vi "Event Messenger Channel Lesson 6.vi"() -> ()   [LabVIEW 2019]
doc: "Lesson 6 is the same messaging system as Lesson 5 but uses a LabVIEW class message hierarchy. This lesson shows the event channels in a form that is highly flexible for a multiple-module system. Its architecture is very similar to the Actor Framework. Channel wires express static connections between parallel systems; AF expresses dynamic connections."
uses:
  <extravilib>/ChannelInstances/Event Messenger-class'Draw Messages.lvlib-Draw Message'/Event Data.ctl
  SubVIs/Draw Messages/Draw Message/Draw Message.lvclass
  <extravilib>/ChannelInstances/Event Messenger-u32/Event Data.ctl
  SubVIs/Draw Messages/Reset Message/Reset Message.lvclass
  e:/builds/penguin/labview/branches/2019/dev/dist/examples/Channels/Event Messenger/SubVIs/Draw Messages/Draw Message/Draw Message.lvclass
  SubVIs/Draw Messages/Square Message/Square Message.lvclass
  SubVIs/Draw Messages/Circle Message/Circle Message.lvclass
  <extravilib>/ChannelInstances/Event Messenger-class'Draw Messages.lvlib-Draw Message'/Instantiate.vi
  <extravilib>/ChannelInstances/Event Messenger-class'Draw Messages.lvlib-Draw Message'/))Channel.vi
  <extravilib>/ChannelInstances/Event Messenger-u32/Instantiate.vi
  <extravilib>/ChannelInstances/Event Messenger-u32/))Channel.vi
  <extravilib>/ChannelInstances/Event Messenger-u32.lvlib
  <extravilib>/ChannelInstances/Event Messenger-class'Draw Messages.lvlib-Draw Message'.lvlib
panel:
  out "Picture":picture
  out "current color":u32(colorbox)
  out "command log":string
  in  "Stop Gamma":bool
  in  "Stop Epsilon":bool
  in  "Stop Beta":bool
  in  "Stop Alpha":bool
  # "Overview: This VI demonstrates how to use the Event Messenger channel wire.\n\nLesson 6 is the same messaging system as Lesson 5 but uses a LabVIEW class message hierarchy. This lesson uses the channels to form a flexible, multiple-module system. Its architecture is very similar to the Actor Framework. Channel wires express static connections between parallel systems; AF expresses dynamic connections.\n\nInstructions:\n1. Run the VI. There are three producers and two consumers, all running at various speeds. Alpha and beta loops produce object commands. Gamma loop produces a color. Delta loop has the job to log all the commands. Epsilon loop actually does the work of the commands and handles color changes. Epsilon also sends commands to itself, which are properly logged by Delta.\n\n2. Stop the VI by pressing any of the STOP buttons. There will be a slight delay until loop Gamma stops because of its 2 second Wait. \n\n3. Open the block diagram. Review the comments there to see how this VI works."
  # "Producers"
  # "Consumers"
  # "Consumer Delta"
  # "Consumer Epsilon"
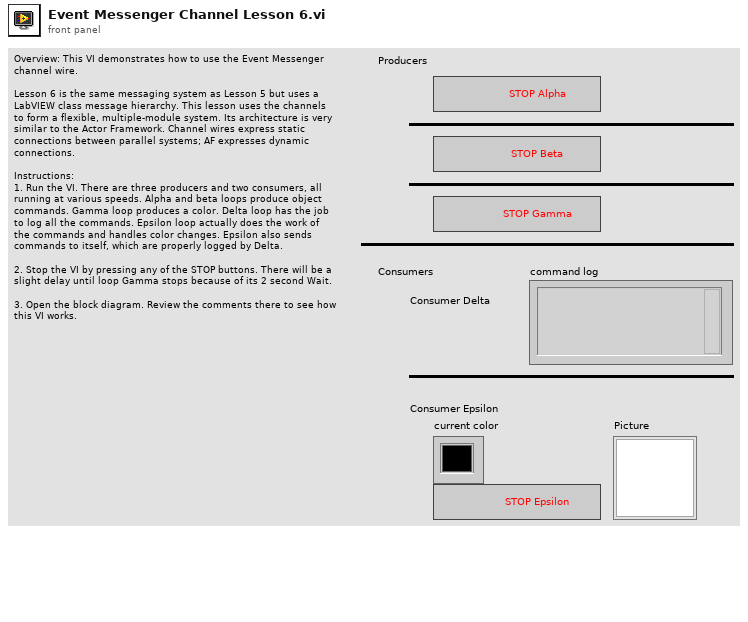
[diagram p1: front panel]
types:
  T1 = cluster{"command":refnum<event-registration>, "new color":refnum<event-registration>}
  T2 = typedef "Event Messenger-class'Draw Messages.lvlib-Draw Message'.lvlib/))Channel.ctl" = refnum<queue>
  T3 = typedef "Event Messenger-u32.lvlib/))Channel.ctl" = refnum<queue>
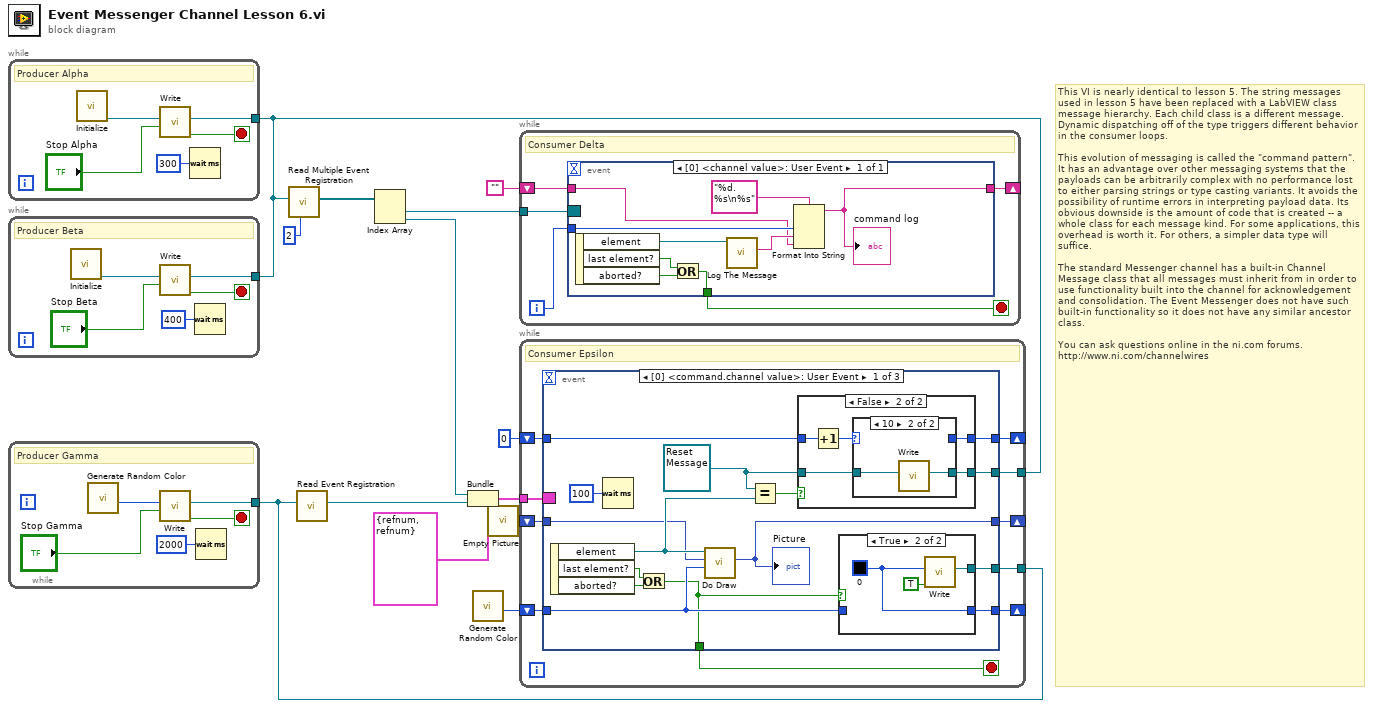
[diagram p0: block diagram]
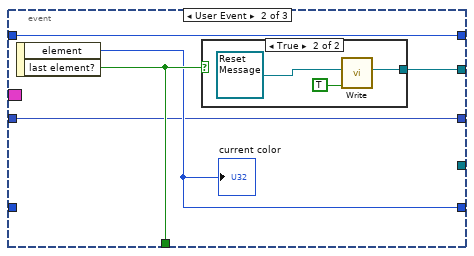
[diagram p5: hidden frame]
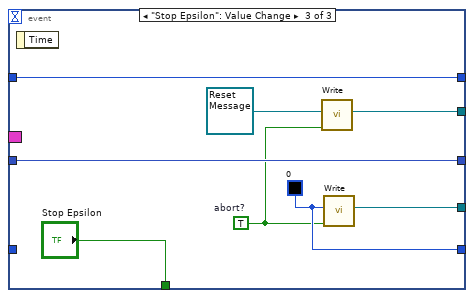
[diagram p7: hidden frame]
diagram:
  # "This VI is nearly identical to lesson 5. The string messages used in lesson 5 have been replaced with a LabVIEW class message hierarchy. Each child class is a different message. Dynamic dispatching off of the type triggers different behavior in the consumer loops.\n\nThis evolution of messaging is called the \"command pattern\". It has an advantage over other messaging systems that the payloads can be arbitrarily complex with no performance lost to either parsing strings or type casting variants. It avoids the possibility of runtime errors in interpreting payload data. Its obvious downside is the amount of code that is created -- a whole class for each message kind. For some applications, this overhead is worth it. For others, a simpler data type will suffice.\n\nThe standard Messenger channel has a built-in Channel Message class that all messages must inherit from in order to use functionality built into the channel for acknowledgement and consolidation. The Event Messenger does not have such built-in functionality so it does not have any similar ancestor class.\n\nYou can ask questions online in the ni.com forums. \nhttp://www.ni.com/channelwires"
  n1 = while {
    tunnel: [w18] -> w2
    stop <- w16 stop-if-true
    # "Producer Alpha"
    n2 = call "Initialize.vi"() -> ("Draw Message"=w14:refnum<class "Draw Message.lvclass">)  [unwired: 11 in]
    n3 = call <extravilib>:"Write.vi"("last element? (F)"="Stop Alpha", "element"=w14) -> ("done?"=w16:bool, "channel"=w18:T2)  [unwired: 8 in]
    n4 = Wait (ms)(milliseconds to wait=u32 300) -> ()  [unwired: 1 out]
  }
  n5 = while {
    tunnel: w2 -> [w21]
    stop <- w22 stop-if-true
    # "Producer Beta"
    n6 = call "Initialize.vi"() -> ("Draw Message"=w19:refnum<class "Draw Message.lvclass">)  [unwired: 7 in]
    n7 = call <extravilib>:"Write.vi"("last element? (F)"="Stop Beta", "element"=w19) -> ("done?"=w22:bool, "channel"=w21:T2)  [unwired: 8 in]
    n8 = Wait (ms)(milliseconds to wait=u32 400) -> ()  [unwired: 1 out]
  }
  n9 = while {
    tunnel: [w26] -> w7
    stop <- w27 stop-if-true
    # "Producer Gamma"
    n10 = call "Generate Random Color.vi"() -> ("Color"=w24:u32)  [unwired: 11 in]
    n11 = call <extravilib>:"Write.vi"("last element? (F)"="Stop Gamma", "element"=w24) -> ("done?"=w27:bool, "channel"=w26:T3)  [unwired: 8 in]
    n12 = Wait (ms)(milliseconds to wait=u32 2000) -> ()  [unwired: 1 out]
  }
  n13 = call <extravilib>:"Read Multiple Event Registration.vi"("number of event structures"=u16 2 ("# Event structures"), "channel"=w2) -> ("event registration refnums"=w10:refnum<event-registration>[])  [unwired: 9 in]
  n14 = call <extravilib>:"Read Event Registration.vi"("channel"=w7) -> ("event registration refnum"=w8:refnum<event-registration>)  [unwired: 10 in]
  n15 = Index Array(array=w10) -> (element #1=w12:refnum<event-registration>, element #2=w11:refnum<event-registration>)  [unwired: 2 in]
  n16 = Bundle(cluster=T1 {"command"=refnum, "new color"=refnum}, "command"=w11, "new color"=w8) -> (w13:T1)
  n17 = call "Generate Random Color.vi"() -> ("Color"=w6:u32)  [unwired: 11 in]
  n18 = call "Empty Picture"() -> ("empty picture"=w3:picture)
  n19 = while {
    tunnel: w12 -> [w33]
    shift-right: [w29] -> _
    shift-left: "" -> [w31]
    i -> [w30]
    stop <- w32 stop-if-true
    # "Consumer Delta"
    n20 = event shown="[0] <channel value>: User Event" {
      selector: w33 -> [_]
      dyn-events: _ -> [_]
      timeout: _ -> [_]
      tunnel: [w34] -> w32
      tunnel: w31 -> [w38]
      tunnel: w30 -> [w40]
      tunnel: [w37] -> w29
      event User Event {
        n21 = event-data() -> ("element"=w42:refnum<class "Draw Message.lvclass">, "last element?"=w35:bool, "aborted?"=w36:bool)  [unwired: 1 in]
        n22 = Or(x=w35, y=w36) -> (x .or. y?=w34:bool)
        n23 = call-dynamic "Log The Message.vi"("Draw Message"=w42) -> ("log text"=w39:string)  [unwired: 10 in]
        n24 = Format Into String(format string="%d. %s\n%s", w40, w39, w38) -> (resulting string=w37:string)  [unwired: 2 in, 1 out]
        "command log" <- w37
      }
    }
  }
  n25 = while {
    tunnel: w13 -> [w51]
    tunnel: w2 -> [w50]
    tunnel: w7 -> [w49]
    shift-right: [w48] -> _
    shift-left: w6 -> [w47]
    shift-right: [w45] -> _
    shift-left: u8 0 -> [w46]
    shift-right: [w44] -> _
    shift-left: w3 -> [w43]
    stop <- w52 stop-if-true
    # "Consumer Epsilon"
    n26 = event shown="[0] <command.channel value>: User Event" {
      selector: w51 -> [_ _ _]
      dyn-events: _ -> [_ _ _]
      timeout: _ -> [_ _ _]
      tunnel: [w53 w84 "Stop Epsilon"] -> w52
      tunnel: [w67 w85 w90] -> w50
      tunnel: [w66 _ w95] -> w49
      tunnel: [w64 w83 w94] -> w48
      tunnel: w47 -> [w56 _ _]
      tunnel: w46 -> [w63 w82 w93]
      tunnel: [w62 w82 w93] -> w45
      tunnel: [w57 w81 w92] -> w44
      tunnel: w43 -> [w58 w81 w92]
      event User Event {
        w60 = refnum<class "Reset Message.lvclass"> refnum ("Draw Messages.lvlib:Circle Message.lvclass")
        n27 = event-data() -> ("element"=w59:refnum<class "Draw Message.lvclass">, "last element?"=w54:bool, "aborted?"=w55:bool)  [unwired: 1 in]
        n28 = Wait (ms)(milliseconds to wait=u32 100) -> ()  [unwired: 1 out]
        n29 = Or(x=w54, y=w55) -> (x .or. y?=w53:bool)
        n30 = call-dynamic "Do Draw.vi"("color"=w56, "picture in"=w58, "Draw Message"=w59) -> ("picture out"=w57:picture)  [unwired: 8 in]
        "Picture" <- w57
        n31 = Equal?(x=w60, y=w59) -> (x = y?=w61:bool)
        n32 = case shown="False" w61 {
          tunnel: [_ w77] -> w67
          tunnel: w63 -> [w72 w76]
          tunnel: [w72 w74] -> w62
          tunnel: w60 -> [_ w73]
          frame True {
          }
          frame False {
            n33 = Increment(x=w76) -> (x+1=w75:u8)
            n34 = case shown="10" w75 {
              selector: w75 -> [w78 _]
              tunnel: [_ w80] -> w77
              tunnel: [w78 _] -> w74
              tunnel: w73 -> [_ w79]
              frame Default {
              }
              frame 10 {
                n35 = call <extravilib>:"Write.vi"("element"=w79) -> ("channel"=w80:T2)  [unwired: 9 in, 1 out]
              }
            }
          }
        }
        n36 = case shown="True" w53 {
          tunnel: [_ w71] -> w66
          tunnel: [w68 w69] -> w64
          tunnel: w56 -> [w68 _]
          frame False {
          }
          frame True {
            w69 = u32 0 ("random color")
            n37 = call <extravilib>:"Write.vi"("abort (F)"=TRUE ("element valid? (T)"), "element"=w69) -> ("channel"=w71:T3)  [unwired: 8 in, 1 out]
          }
        }
      }
      event User Event {
        n38 = event-data() -> ("element"=w83:u32, "last element?"=w84:bool)  [unwired: 1 in]
        "current color" <- w83
        n39 = case shown="True" w84 {
          tunnel: [_ w88] -> w85
          frame False {
          }
          frame True {
            n40 = call <extravilib>:"Write.vi"("abort (F)"=TRUE ("element valid? (T)"), "element"=refnum<class "Reset Message.lvclass"> refnum ("Draw Messages.lvlib:Reset Message.lvclass")) -> ("channel"=w88:T2)  [unwired: 8 in, 1 out]
          }
        }
      }
      event "Stop Epsilon": Value Change {
        w94 = u32 0 ("random color")
        w89 = TRUE  # abort?
        n41 = event-data() -> ()  [unwired: 1 in, 1 out]
        n42 = call <extravilib>:"Write.vi"("abort (F)"=w89, "element"=refnum<class "Reset Message.lvclass"> refnum ("Draw Messages.lvlib:Reset Message.lvclass")) -> ("channel"=w90:T2)  [unwired: 8 in, 1 out]
        n43 = call <extravilib>:"Write.vi"("abort (F)"=w89, "element"=w94) -> ("channel"=w95:T3)  [unwired: 8 in, 1 out]
      }
    }
  }
